vi "Write.vi"(7 "Input String":string, 8 "error in (no error)":errorcluster, 11 "VISA resource name":refnum<visa-resource-name>) -> (0 "error out":errorcluster, 2 "String":string, 3 "VISA resource name out":refnum<visa-resource-name>)   [LabVIEW 2022 SP3, in "BK Precision 9103.lvlib"]
doc: "Performs a VISA write operation with an added delay to allow additional time for instrument to process."
uses:
  <instrlib>/BK Precision 9103/BK Precision 9103.lvlib
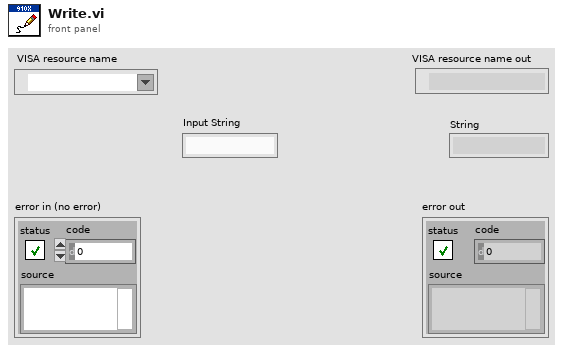
[diagram p1: front panel]
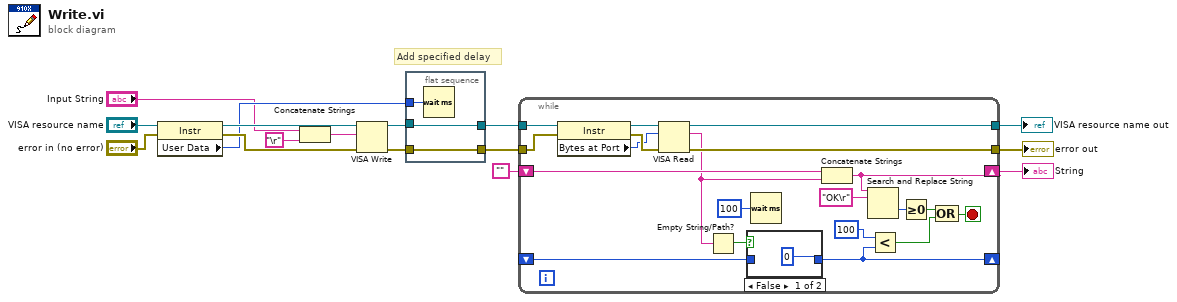
[diagram p0: block diagram]
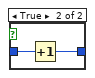
[diagram p2: hidden frame]
diagram:
  # "Add specified delay"
  n1 = property class="Instr"(reference="VISA resource name", error in="error in (no error)") -> (reference out=w14:refnum<visa-resource-name>, error out=w13:errorcluster, "User Data"=w12:u32)
  n2 = Concatenate Strings("Input String", "\r") -> (w9:string)
  n3 = VISA Write(VISA resource name=w14, write buffer=w9, error in (no error)=w13) -> (VISA resource name out=w11:refnum<visa-resource-name>, error out=w10:errorcluster)  [unwired: 1 out]
  n4 = flat-sequence {
    tunnel: w12 -> [w19]
    tunnel: w11 -> [w18]
    tunnel: [w18] -> w5
    tunnel: w10 -> [w17]
    tunnel: [w17] -> w6
    frame #0 {
      n5 = Wait (ms)(milliseconds to wait=w19) -> ()  [unwired: 1 out]
    }
  }
  n6 = while {
    tunnel: [w39] -> w4
    shift-right: [w36] -> w2
    shift-left: "" -> [w38]
    shift-right: [w30] -> _
    shift-left: _ -> [w31]
    tunnel: w5 -> [w24]
    tunnel: w6 -> [w22]
    tunnel: [w27] -> w3
    stop <- w37 stop-if-true
    n7 = property class="Instr"(reference=w24, error in=w22) -> (reference out=w23:refnum<visa-resource-name>, error out=w21:errorcluster, "Bytes at Port"=w20:u32)
    n8 = VISA Read(VISA resource name=w23, byte count=w20, error in (no error)=w21) -> (VISA resource name out=w39:refnum<visa-resource-name>, read buffer=w26:string, error out=w27:errorcluster)  [unwired: 1 out]
    n9 = Empty String/Path?(string/path=w26) -> (empty?=w32:bool)
    n10 = case shown="False" w32 {
      tunnel: w31 -> [_ w42]
      tunnel: [0 w41] -> w30
      frame False {
      }
      frame True {
        n11 = Increment(x=w42) -> (x+1=w41:i32)
      }
    }
    n12 = Wait (ms)(milliseconds to wait=u32 100) -> ()  [unwired: 1 out]
    n13 = Concatenate Strings(w38, w26) -> (w36:string)
    n14 = Search and Replace String(input string=w36, search string="OK\r" ("y")) -> (offset past replacement=w34:i32)  [unwired: 6 in, 3 out]
    n15 = Less?(x=100, y=w30) -> (x < y?=w28:bool)
    n16 = Greater Or Equal To 0?(x=w34) -> (x >= 0?=w33:bool)
    n17 = Compound Arithmetic op=OR(w33, w28) -> (w37:bool)
  }
  "error out" <- w3
  "VISA resource name out" <- w4
  "String" <- w2
